vi "Logging Names.vi"() -> (0 "error out":errorcluster, 1 "Name Cluster":T1, 2 "FIFO Cluster":T2)   [LabVIEW 2017]
uses:
  Controls/Logging names.ctl
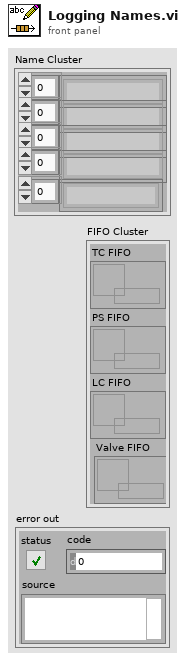
[diagram p1: front panel]
types:
  T1 = typedef "Logging names.ctl" = cluster{"Keys":string[], "TC Names":string[], "PC Names":string[], "LC Names":string[], "Valve Names":string[]}
  T2 = cluster{"TC FIFO":refnum<k33>, "PS FIFO":refnum<k33>, "LC FIFO":refnum<k33>, "Valve FIFO":refnum<k33>}
  T3 = cluster{"rt fifo":refnum<k33>, "rt fifo":refnum<k33>, "rt fifo":refnum<k33>, "rt fifo 2":refnum<k33>}
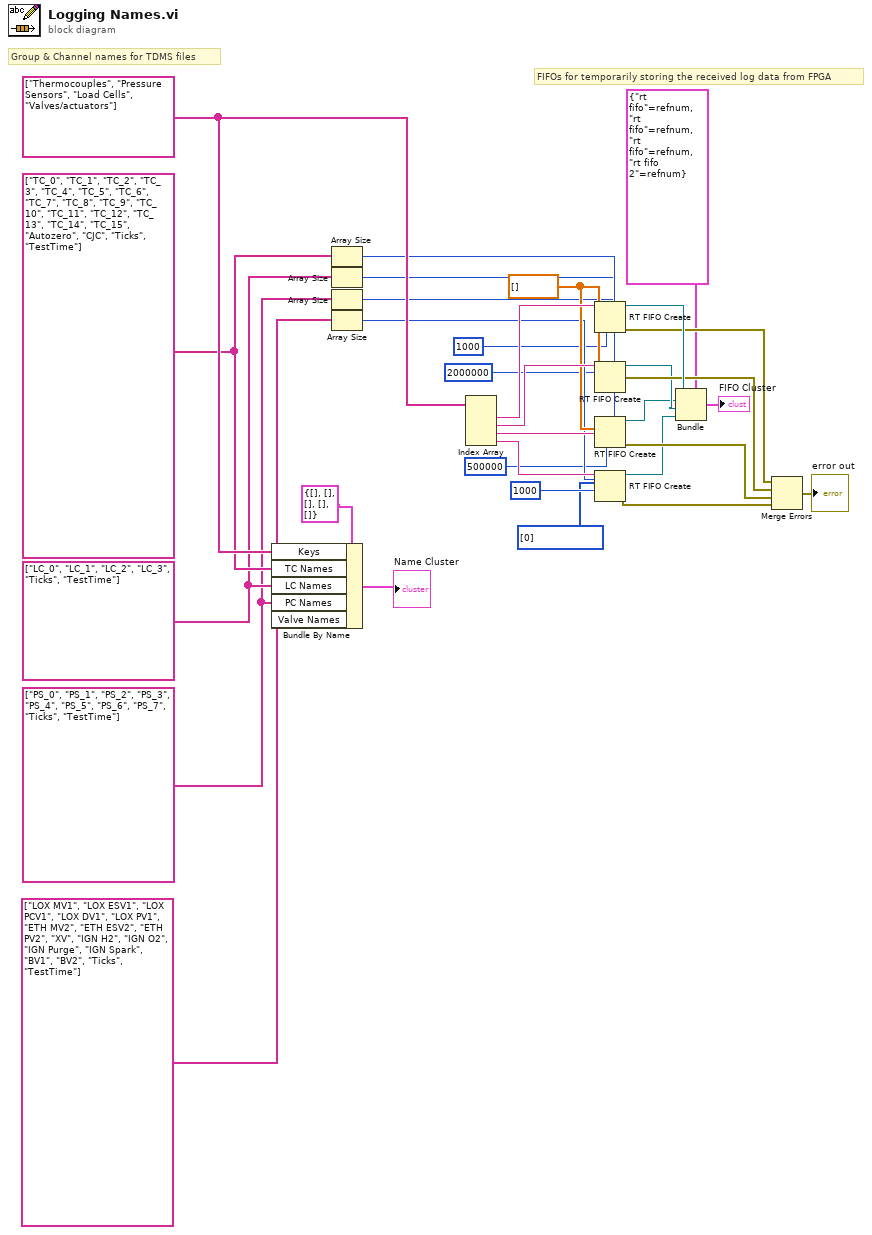
[diagram p0: block diagram]
diagram:
  w27 = sgl[] []
  w19 = string[] ["LOX MV1", "LOX ESV1", "LOX PCV1", "LOX DV1", "LOX PV1", "ETH MV2", "ETH ESV2", "ETH PV2", "XV", "IGN H2", "IGN O2", "IGN Purge", "IGN Spark", "BV1", "BV2", "Ticks", "TestTime"]
  w22 = string[] ["TC_0", "TC_1", "TC_2", "TC_3", "TC_4", "TC_5", "TC_6", "TC_7", "TC_8", "TC_9", "TC_10", "TC_11", "TC_12", "TC_13", "TC_14", "TC_15", "Autozero", "CJC", "Ticks", "TestTime"]
  w21 = string[] ["LC_0", "LC_1", "LC_2", "LC_3", "Ticks", "TestTime"]
  w20 = string[] ["PS_0", "PS_1", "PS_2", "PS_3", "PS_4", "PS_5", "PS_6", "PS_7", "Ticks", "TestTime"]
  w32 = string[] ["Thermocouples", "Pressure Sensors", "Load Cells", "Valves/actuators"]
  # "FIFOs for temporarily storing the received log data from FPGA"
  # "Group & Channel names for TDMS files"
  n1 = Bundle By Name(cluster=T1 {"Keys"=[], "TC Names"=[], "PC Names"=[], "LC Names"=[], "Valve Names"=[]} ("input cluster"), "Keys"=w32, "TC Names"=w22, "LC Names"=w21, "PC Names"=w20, "Valve Names"=w19) -> (→"Name Cluster":T1)
  n2 = Array Size(array=w22) -> (size(s)=w26:i32)
  n3 = Array Size(array=w21) -> (size(s)=w25:i32)
  n4 = Array Size(array=w20) -> (size(s)=w24:i32)
  n5 = Array Size(array=w19) -> (size(s)=w23:i32)
  n6 = Index Array(array=w32) -> (element #1=w31:string, element #2=w30:string, element #3=w29:string, element #4=w28:string)  [unwired: 4 in]
  n7 = RT FIFO Create(0:w31, 1:w27, 4:u32 1000 ("size (10)"), 6:w26) -> (8:w13:refnum<k33>, 11:w12:errorcluster)  [unwired: 4 in, 1 out]
  n8 = RT FIFO Create(0:w30, 1:w27, 4:u32 2000000 ("size (10)"), 6:w25) -> (8:w4:refnum<k33>, 11:w11:errorcluster)  [unwired: 4 in, 1 out]
  n9 = RT FIFO Create(0:w29, 1:w27, 4:u32 500000 ("size (10)"), 6:w24) -> (8:w3:refnum<k33>, 11:w10:errorcluster)  [unwired: 4 in, 1 out]
  n10 = RT FIFO Create(0:w28, 1:i32[] [0], 4:u32 1000 ("size (10)"), 6:w23) -> (8:w6:refnum<k33>, 11:w9:errorcluster)  [unwired: 4 in, 1 out]
  n11 = Bundle(cluster=T3 {"rt fifo"=refnum, "rt fifo"=refnum, "rt fifo"=refnum, "rt fifo 2"=refnum}, "rt fifo"=w13, "rt fifo"=w3, "rt fifo"=w4, "rt fifo 2"=w6) -> (→"FIFO Cluster":T3)
  n12 = Merge Errors(w12, w11, w10, w9) -> (→"error out":errorcluster)
